vi "Decode Status Byte.vi"(2 "Window Mode Notifier":refnum<notifier>, 3 "Status":T1) -> (0 "Status":T3(ring), 1 "Mode":T2(ring)=enum."Auto Disabled")   [LabVIEW 2014]
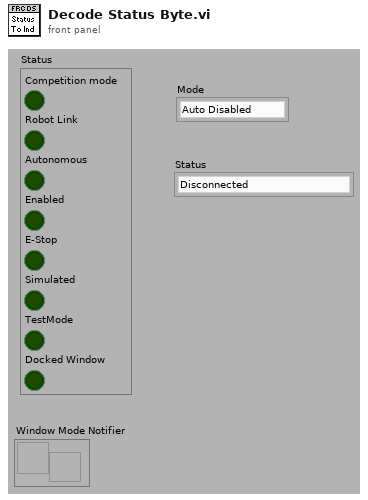
[diagram p1: front panel]
types:
  T1 = cluster{"Competition mode":bool, "Robot Link":bool, "Autonomous":bool, "Enabled":bool, "E-Stop":bool, "Simulated":bool, "TestMode":bool, "Docked Window":bool}
  T2 = enum8{"Tele-Op Disabled", "Tele-Op Enabled", "Auto Disabled", "Auto Enabled", "Test Disabled", "Test Enabled", ""}
  T3 = enum8{"Disconnected", "E-Stop", "Disabled", "Enabled"}
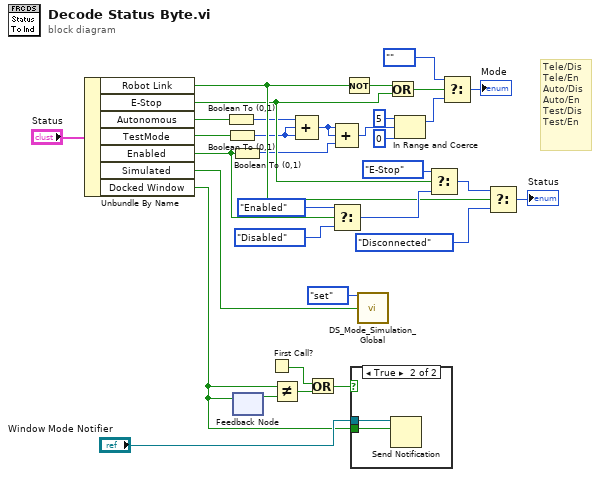
[diagram p0: block diagram]
diagram:
  # "Tele/Dis\nTele/En\nAuto/Dis\nAuto/En\nTest/Dis\nTest/En"
  n1 = Unbundle By Name("Status") -> ("Robot Link"=w26:bool, "E-Stop"=w20:bool, "Autonomous"=w23:bool, "TestMode"=w19:bool, "Enabled"=w5:bool, "Simulated"=w6:bool, "Docked Window"=w9:bool)
  n2 = Boolean To (0,1)(Boolean=w23) -> (0, 1=w18:i16)
  n3 = Boolean To (0,1)(Boolean=w19) -> (0, 1=w17:i16)
  n4 = Boolean To (0,1)(Boolean=w5) -> (0, 1=w2:i16)
  n5 = feedback-in #1(w9) -> ()
  n6 = feedback #1() -> (w13:bool)  [unwired: 1 in]
  n7 = First Call?() -> (First Call?: T/F=w11:bool)
  n8 = Not Equal?(x=w9, y=w13) -> (x != y?=w12:bool)
  n9 = Compound Arithmetic op=ADD(w18, w17, w17) -> (w3:i16)
  n10 = Or(x=w11, y=w12) -> (x .or. y?=w8:bool)
  n11 = Select(t=T3."Enabled" ("Status"), s=w5, f=T3."Disabled" ("Status")) -> (s? t:f=w31:T3)
  n12 = Compound Arithmetic op=ADD(w3, w3, w2) -> (w4:i16)
  n13 = Not(x=w26) -> (.not. x?=w22:bool)
  n14 = case shown="True" w8 {
    tunnel: "Window Mode Notifier" -> [_ w35]
    tunnel: w9 -> [_ w34]
    frame False {
    }
    frame True {
      n15 = Send Notification(notification=w34, notifier=w35) -> ()  [unwired: 1 in, 2 out]
    }
  }
  n16 = call <vilib>:"DS_Mode_Simulation_Global.vi"("menu"=enum16{"set", "get"}."set", "simulated? in"=w6) -> ()  [unwired: 12 in, 2 out]
  n17 = Or(x=w22, y=w20) -> (x .or. y?=w24:bool)
  n18 = In Range and Coerce(upper limit=i16 5, x=w4, lower limit=i16 0) -> (coerced(x)=w14:i16)  [unwired: 1 out]
  n19 = Select(t=T3."E-Stop" ("Status"), s=w20, f=w31) -> (s? t:f=w29:T3)
  n20 = Select(t=T2."" ("Mode"), s=w24, f=w14) -> (s? t:f=→"Mode":i16)
  n21 = Select(t=w29, s=w26, f=T3."Disconnected" ("Status")) -> (s? t:f=→"Status":T3)
